vi "Write timestamp.vi"(8 "error in (no error)":errorcluster, 10 "timestamp":timestamp format="%<%x %.3X>T", 11 "syslogs in":refnum<class "syslogs.lvclass">) -> (0 "error out":errorcluster, 3 "syslogs out":refnum<class "syslogs.lvclass">)   [LabVIEW 2020, in "ORM_Examples.lvlib" / "syslogs.lvclass"]
uses:
  syslogs.lvclass
  syslogs.lvclass/syslogs.ctl
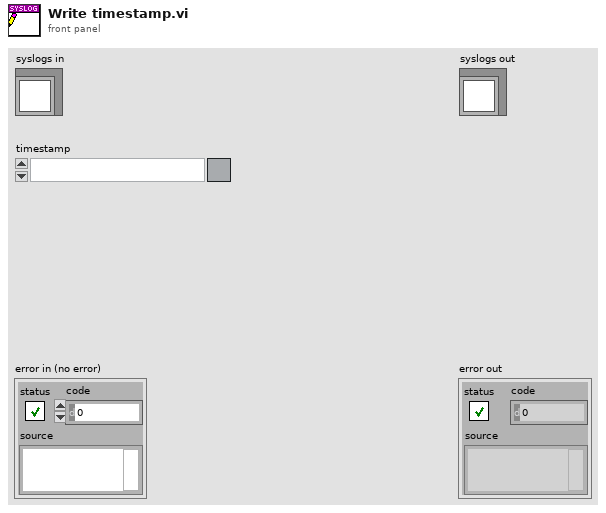
[diagram p1: front panel]
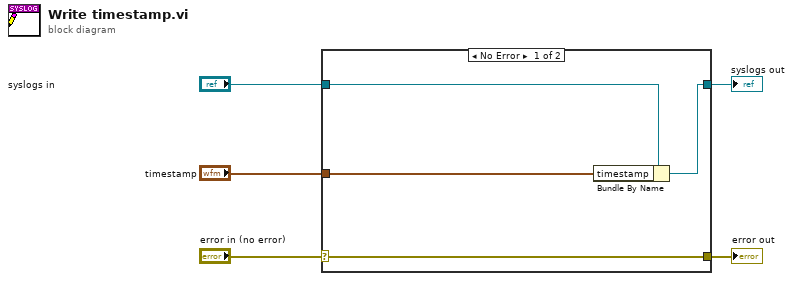
[diagram p0: block diagram]
diagram:
  n1 = case shown="No Error" "error in (no error)" {
    selector: "error in (no error)" -> [w9 w10]
    tunnel: [w9 w10] -> w4
    tunnel: [w7 w11] -> w2
    tunnel: "syslogs in" -> [w8 w11]
    tunnel: "timestamp" -> [w6 _]
    frame No Error {
      n2 = Bundle By Name(cluster=w8, "timestamp"=w6) -> (w7:refnum<class "syslogs.lvclass">)
    }
    frame Error {
    }
  }
  "error out" <- w4
  "syslogs out" <- w2
